vi "Waveform_Extract from Start and End time with End point.vi"(8 "Error":errorcluster, 9 "End Time":dbl, 10 "Begin Time":dbl, 11 "Waveform":T1) -> (0 "Error Out":errorcluster, 1 "End Index Out":i32, 2 "Start Index Out":i32, 3 "Waveform Out":T1)   [LabVIEW 2024]
doc: "Retrieves a subset of a waveform at a specified time or index. You must manually select the polymorphic instance you want to use."
uses:
  Universal Controls/Waveform_Data.ctl
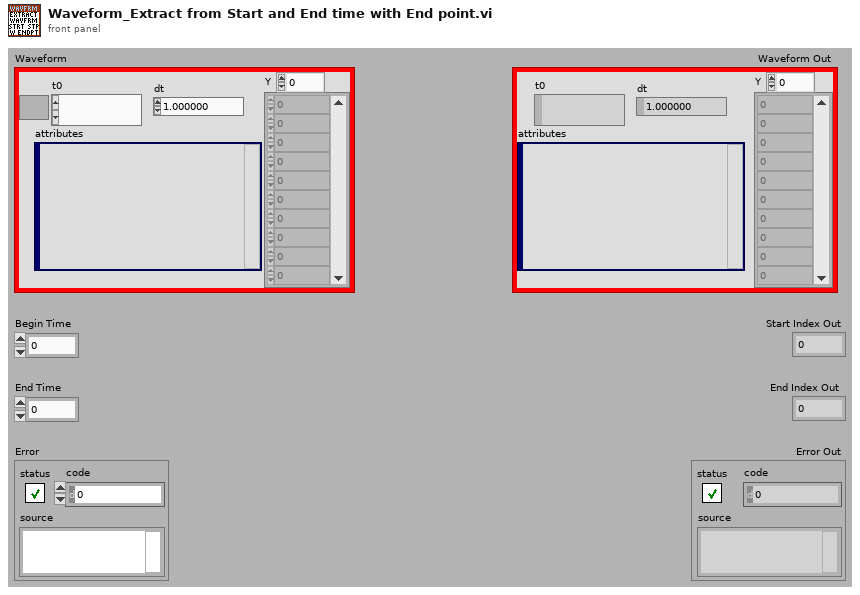
[diagram p1: front panel]
types:
  T1 = typedef "Waveform_Data.ctl" = waveform(dbl)
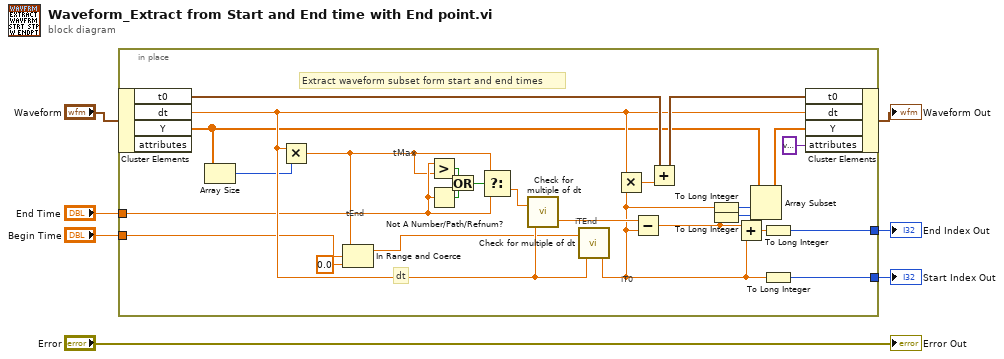
[diagram p0: block diagram]
diagram:
  n1 = in-place {
    in-place-border: "Begin Time" -> [w12]
    in-place-border: "End Time" -> [w17]
    in-place-border: [w28] -> w5
    in-place-border: [w27] -> w4
    # "Extract waveform subset form start and end times"
    # "dt"
    # "iTEnd"
    # "iT0"
    # "tEnd"
    # "tMax"
    n2 = in-place-cluster #1("Waveform") -> ("t0"=w20:timestamp, "dt"=w18:dbl, "Y"=w9:dbl[])  [unwired: 1 out]
    n3 = Array Size(array=w9) -> (size(s)=w8:i32)
    n4 = Multiply(x=w18, y=w8) -> (x*y=w14:dbl)
    n5 = In Range and Coerce(upper limit=w14, x=w12, lower limit=0.0) -> (coerced(x)=w11:dbl)  [unwired: 1 out]
    n6 = Greater?(x=w17, y=w14) -> (0:w32:bool)
    n7 = Not A Number/Path/Refnum?(number/path/refnum=w17) -> (NaN/Path/Refnum?=w31:bool)
    n8 = Or(x=w32, y=w31) -> (x .or. y?=w30:bool)
    n9 = Select(t=w14, s=w30, f=w17) -> (s? t:f=w15:dbl)
    n10 = call <vilib>:"Check for multiple of dt.vi"("dt"=w18, "time"=w15) -> ("iQuotient"=w29:dbl)  [unwired: 1 out]
    n11 = call <vilib>:"Check for multiple of dt.vi"("dt"=w18, "time"=w11) -> ("iQuotient"=w26:dbl)  [unwired: 1 out]
    n12 = Multiply(x=w18, y=w26) -> (x*y=w24:dbl)
    n13 = Subtract(x=w29, y=w26) -> (x-y=w16:dbl)
    n14 = Add(x=w20, y=w24) -> (x+y=w19:timestamp)
    n15 = To Long Integer(number=w26) -> (32bit integer=w22:i32)
    n16 = To Long Integer(number=w16) -> (32bit integer=w23:i32)
    n17 = Add(x=w16, y=w26) -> (x+y=w25:dbl)
    n18 = Array Subset(array=w9, index=w22, length=w23) -> (w21:dbl[])
    n19 = To Long Integer(number=w25) -> (32bit integer=w27:i32)
    n20 = To Long Integer(number=w26) -> (32bit integer=w28:i32)
    n21 = in-place-cluster #1("t0"=w19, "dt"=w18, "Y"=w21, "attributes"=variant) -> (→"Waveform Out":T1)
  }
  "Start Index Out" <- w5
  "End Index Out" <- w4
  "Error Out" <- "Error"
